vi "Reset-All-Action_Api.vi"(8 "Error In":errorcluster) -> (0 "Error Out":errorcluster, 2 "I2C Ref Out":T1={"myRIO Reference"={"myRIO Model"=enum."Unknown", "myRIO Hardware Reference"={"Generic FPGA Reference"=refnum, "Allow multiple opens"=FALSE}}, "I2C Channels Enum"=enum."Not Connected", "I2C Configuration"={"I2C Transfer Rate"=enum."Fast mode (400 kbps)"}}, 3 "HiTechnicColorSensorV2 Ref Out":cluster{"I2C Ref Out":T1})   [LabVIEW 2019]
uses:
  <vilib>/myRIO/Instrument Drivers/Onboard IO/I2C/typedefs/I2C Reference.ctl
  <vilib>/myRIO/Common/Instrument Driver Framework/Utilities/typedefs/myRIO Generic Hardware Reference.ctl
  <vilib>/myRIO/Common/Instrument Driver Framework/Utilities/typedefs/Hardware Version Enum.ctl
  <vilib>/myRIO/Common/Instrument Driver Framework/Utilities/typedefs/myRIO v1.0 Reference.ctl
  <vilib>/myRIO/Common/Instrument Driver Framework/Utilities/typedefs/Generic FPGA Reference.ctl
  <vilib>/myRIO/Common/Instrument Driver Framework/myRIO v1.0/I2C/typedefs/I2C Channels Enum.ctl
  <vilib>/myRIO/Instrument Drivers/Onboard IO/I2C/typedefs/I2C Configuration.ctl
  <vilib>/myRIO/Instrument Drivers/Onboard IO/I2C/typedefs/I2C Transfer Rate.ctl
  Variable/Position.vi
  <vilib>/myRIO/Instrument Drivers/Onboard IO/I2C/I2C.lvlib
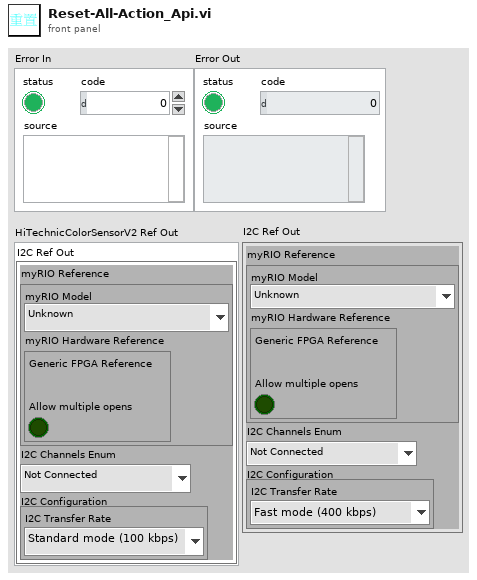
[diagram p1: front panel]
types:
  T1 = typedef "I2C.lvlib/I2C Reference.ctl" = cluster{"myRIO Reference":T2, "I2C Channels Enum":T6, "I2C Configuration":T7}
  T2 = typedef "myRIO Generic Hardware Reference.ctl" = cluster{"myRIO Model":T3, "myRIO Hardware Reference":T4}
  T3 = typedef "Hardware Version Enum.ctl" = enum16{"Unknown", "myRIO-1900", "myRIO-1950", "roboRIO", "NI ELVIS RIO CM", "ELVIS III"}
  T4 = typedef "myRIO v1.0 Reference.ctl" = cluster{"Generic FPGA Reference":T5, "Allow multiple opens":bool}
  T5 = typedef "Generic FPGA Reference.ctl" = refnum<k20>
  T6 = typedef "I2C Channels Enum.ctl" = enum16{"Not Connected", "A/I2C", "B/I2C", "I2C/I2C"}
  T7 = typedef "I2C.lvlib/I2C Configuration.ctl" = cluster{"I2C Transfer Rate":T8}
  T8 = typedef "I2C.lvlib/I2C Transfer Rate.ctl" = enum16{"Standard mode (100 kbps)", "Fast mode (400 kbps)"}
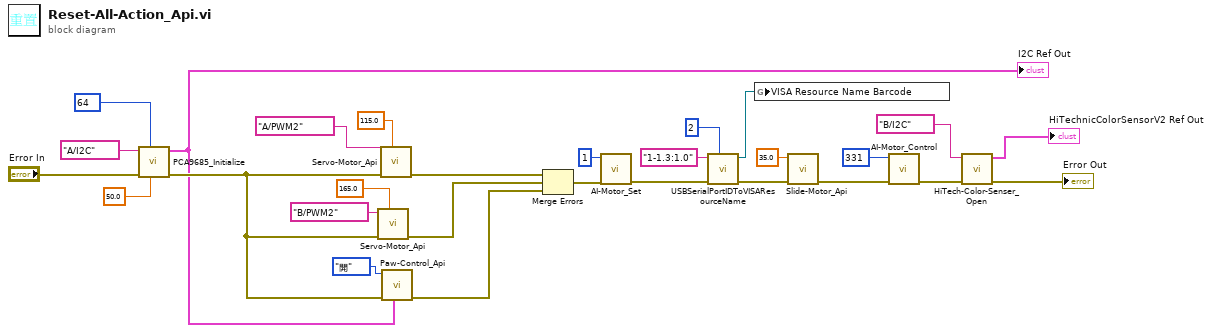
[diagram p0: block diagram]
diagram:
  n1 = call "PCA9685_Initialize.vi"("PWM頻率(50Hz)"=50.0, "驅動板位址(0x40)"=u8 64, "Error In"="Error In", "I2C腳位"=tag "A/I2C") -> ("Error Out"=w21:errorcluster, "I2C Ref Out"=w17:T1)  [unwired: 6 in]
  "I2C Ref Out" <- w17
  n2 = call "Servo-Motor_Api.vi"("角度"=165.0, "Error In"=w21, "伺服馬達角位"=tag "B/PWM2") -> ("Error Out"=w28:errorcluster)  [unwired: 8 in]
  n3 = call "Servo-Motor_Api.vi"("角度"=115.0, "Error In"=w21, "伺服馬達角位"=tag "A/PWM2") -> ("Error Out"=w25:errorcluster)  [unwired: 8 in]
  n4 = call "Paw-Control_Api.vi"("I2C Ref In"=w17, "Error In"=w21, "夾爪動作"=enum16{"開", "合"}."開") -> ("error out"=w20:errorcluster)  [unwired: 8 in]
  n5 = Merge Errors(w25, w28, w20) -> (w7:errorcluster)
  n6 = call "AI-Motor_Set.vi"("Error In"=w7, "Motor ID (0)"=u8 1) -> ("Error Out"=w4:errorcluster)  [unwired: 9 in]
  n7 = call "USBSerialPortIDToVISAResourceName.vi"("搜索有效數量"=u32 2, "Error In"=w4, "端口號"="1-1.3:1.0") -> ("Error Out"=w5:errorcluster, "VISA Resource Name"=w2:refnum<visa-resource-name>)  [unwired: 7 in]
  n8 = global write "Position.vi" "VISA Resource Name Barcode"(w2) -> ()
  n9 = call "Slide-Motor_Api.vi"("Error In"=w5, "移動距離"=35.0) -> ("Error Out"=w12:errorcluster)  [unwired: 9 in]
  n10 = call "AI-Motor_Control.vi"("Error In"=w12, "目標位置(0~4095)"=u16 331) -> ("Error Out"=w11:errorcluster)  [unwired: 9 in]
  n11 = call "HiTech-Color-Senser_Open.vi"("Error In"=w11, "I2C角位"=tag "B/I2C") -> ("Error Out"=→"Error Out":errorcluster, "HiTechnicColorSensorV2 Ref Out"=→"HiTechnicColorSensorV2 Ref Out":cluster{"I2C Ref Out":T1})  [unwired: 8 in]
